vi "Wait on Listener.vi"(8 "error in (no error)":errorcluster, 9 "timeout ms (5000)":i32=5000, 11 "VISA TCP Listener in":refnum<class "VISA TCP Listener.lvclass">) -> (0 "error out":errorcluster, 2 "Socket out":refnum<class "Socket.lvclass">, 3 "VISA TCP Listener out":refnum<class "VISA TCP Listener.lvclass">)   [LabVIEW 2013, in "Sockets.lvlib" / "VISA TCP Listener.lvclass"]
doc: "Listens for an incoming TCP socket connection on the given port."
uses:
  VISA TCP Listener.lvclass
  Socket/Socket.lvclass
  VISA TCP Listener.lvclass/VISA TCP Listener.ctl
  VISA TCP Socket/VISA TCP.lvclass
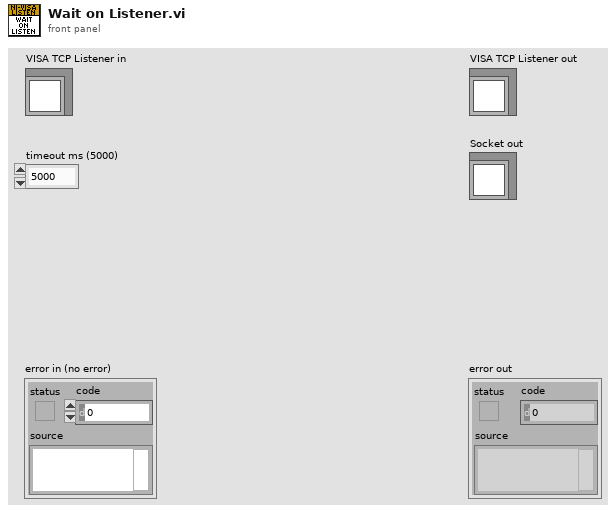
[diagram p1: front panel]
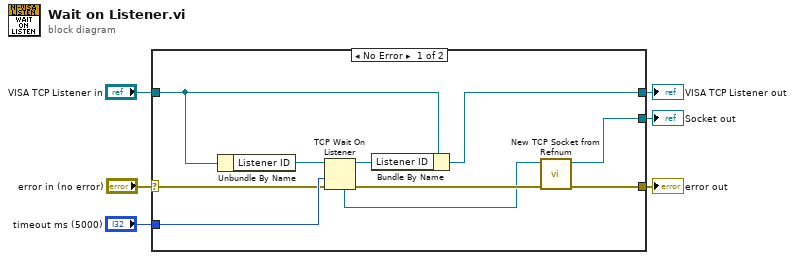
[diagram p0: block diagram]
diagram:
  n1 = case shown="No Error" "error in (no error)" {
    selector: "error in (no error)" -> [w7 w18]
    tunnel: "timeout ms (5000)" -> [w13 _]
    tunnel: [w12 _] -> w5
    tunnel: [w11 w18] -> w4
    tunnel: "VISA TCP Listener in" -> [w9 w17]
    tunnel: [w8 w17] -> w2
    frame No Error {
      n2 = Unbundle By Name(w9) -> ("Listener ID"=w14:refnum<k5>)
      n3 = TCP Wait On Listener(8:w7, 9:w13, 11:w14) -> (0:w16:errorcluster, 3:w10:refnum<k5>, 4:w15:refnum<k5>)  [unwired: 1 in, 2 out]
      n4 = Bundle By Name(cluster=w9, "Listener ID"=w10) -> (w8:refnum<class "VISA TCP Listener.lvclass">)
      n5 = call "New TCP Socket from Refnum.vi"("error in (no error)"=w16, "TCP Network Connection Refnum"=w15) -> ("error out"=w11:errorcluster, "VISA TCP out"=w12:refnum<class "VISA TCP.lvclass">)  [unwired: 8 in]
    }
    frame Error {
    }
  }
  "error out" <- w4
  "VISA TCP Listener out" <- w2
  "Socket out" <- w5
